vi "Top Level Launcher.vi"(6 "Variant in":variant, 7 "Shift Pressed?":bool, 8 "error in":errorcluster, 10 "QD Combo Box Ref":refnum<vi>, 11 "QD Launch VI Ref":refnum<vi>) -> (0 "error out":errorcluster, 4 "Variant out":variant)   [LabVIEW 2020]
doc: "Manages the top level VI in the project.\n\nNormal Operation:\nTo set the top VI, enter \"<b>s</b>\" or \"<b>set</b>\" before activating the shortcut.\nTo open the top VI, use Shift+Ctrl+[shortcut].\nTo run the top VI, use Ctrl+[shortcut].\n\nAdvanced Operation using QD data entry:\nTo run the top VI, enter \"r\" or \"run\" before activating the shortcut.\nTo remove the top VI setting, enter \"d\", \"del\", \"delete\", \"rem\", or \"remove\" before activating the shortcut.\nTo read what the top VI is, enter \"get\" or \"read\" before activating the shortcut.\nTo open the top VI without running it, enter \"o\" or \"open\" before activating the shortcut.\n\nDefault Shortcut - [E]"
panel:
  in  "Undo Name":string="Quick Drop Keyboard Shortcut"
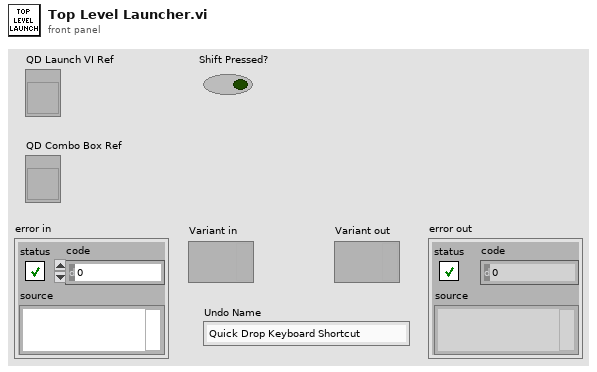
[diagram p1: front panel]
types:
  T1 = typedef "Command Enum.ctl" = enum16{"Invalid", "Invalid Alias", "Run", "Set", "Open", "Read", "Remove"}
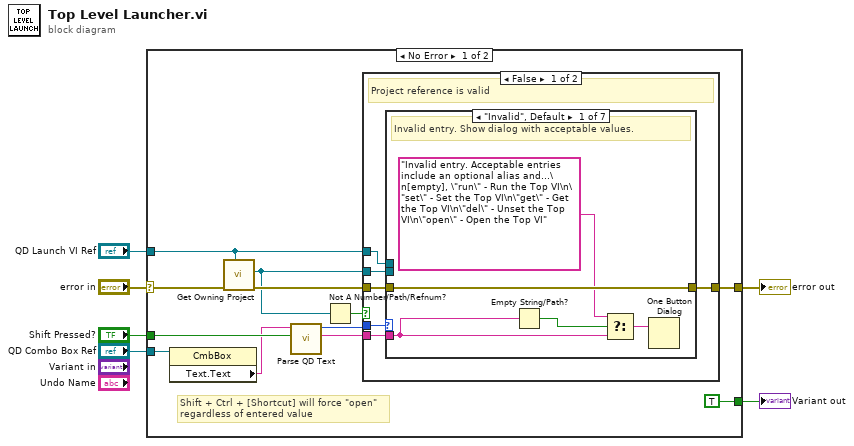
[diagram p0: block diagram]
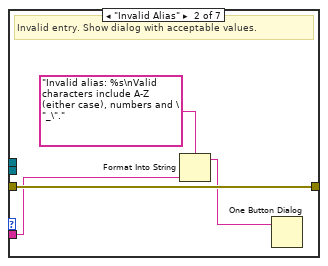
[diagram p2: hidden frame]
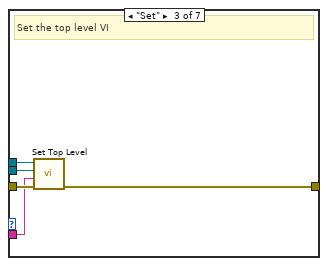
[diagram p3: hidden frame]
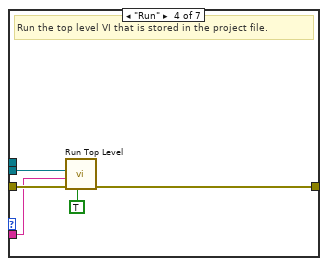
[diagram p4: hidden frame]
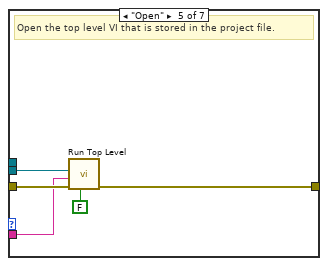
[diagram p5: hidden frame]
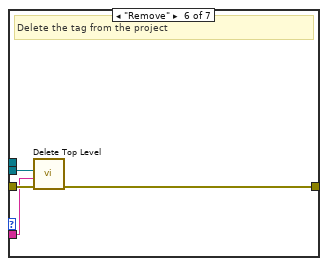
[diagram p6: hidden frame]
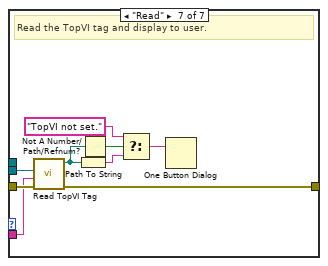
[diagram p7: hidden frame]
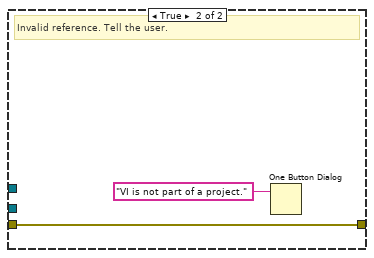
[diagram p8: hidden frame]
diagram:
  n1 = case shown="No Error" "error in" {
    selector: "error in" -> [w17 w64]
    tunnel: [w18 w64] -> w5
    tunnel: "QD Launch VI Ref" -> [w11 _]
    tunnel: "Shift Pressed?" -> [w9 _]
    tunnel: [TRUE _] -> w2
    tunnel: "QD Combo Box Ref" -> [w13 _]
    frame No Error {
      # "Shift + Ctrl + [Shortcut] will force \"open\"\nregardless of entered value"
      n2 = property class="CmbBox"(reference=w13) -> ("Text.Text"=w8:string)  [unwired: 1 in, 2 out]
      n3 = call "Get Owning Project.vi"("VI"=w11, "error in"=w17) -> ("error out"=w16:errorcluster, "Owning Project"=w12:refnum<vi>)  [unwired: 8 in]
      n4 = call "Parse QD Text.vi"("Shift Pressed?"=w9, "QD Combo Box Text"=w8) -> ("Parameter"=w7:string, "Command"=w10:T1)  [unwired: 8 in]
      n5 = Not A Number/Path/Refnum?(number/path/refnum=w12) -> (NaN/Path/Refnum?=w14:bool)
      n6 = case shown="False" w14 {
        tunnel: w10 -> [w22 _]
        tunnel: [w24 w63] -> w18
        tunnel: w16 -> [w23 w63]
        tunnel: w11 -> [w21 _]
        tunnel: w12 -> [w20 _]
        tunnel: w7 -> [w19 _]
        frame False {
          # "Project reference is valid"
          n7 = case shown="\"Invalid\", Default" w22 {
            tunnel: w23 -> [w29 w33 w38 w42 w47 w52 w61]
            tunnel: [w29 w33 w37 w43 w48 w51 w60] -> w24
            tunnel: w21 -> [_ _ w36 _ _ _ _]
            tunnel: w20 -> [_ _ w35 w41 w46 w50 w59]
            tunnel: w19 -> [w26 w31 w34 w39 w44 w49 w53]
            frame "Invalid", Default {
              # "Invalid entry. Show dialog with acceptable values."
              n8 = Empty String/Path?(string/path=w26) -> (empty?=w28:bool)
              n9 = Select(t="Invalid entry. Acceptable entries include an optional alias and...\n[empty], \"run\" - Run the Top VI\n\"set\" - Set the Top VI\n\"get\" - Get the Top VI\n\"del\" - Unset the Top VI\n\"open\" - Open the Top VI" ("message"), s=w28, f=w26) -> (s? t:f=w25:string)
              n10 = One Button Dialog(message=w25) -> ()  [unwired: 1 in, 1 out]
            }
            frame "Invalid Alias" {
              # "Invalid entry. Show dialog with acceptable values."
              n11 = Format Into String(format string="Invalid alias: %s\nValid characters include A-Z (either case), numbers and \"_\"." ("message"), w31) -> (resulting string=w30:string)  [unwired: 2 in, 1 out]
              n12 = One Button Dialog(message=w30) -> ()  [unwired: 1 in, 1 out]
            }
            frame "Set" {
              # "Set the top level VI"
              n13 = call "Set Top Level.vi"("error in"=w38, "Alias"=w34, "Project Reference"=w35, "VI Reference"=w36) -> ("error out"=w37:errorcluster)  [unwired: 7 in]
            }
            frame "Run" {
              # "Run the top level VI that is stored in the project file."
              n14 = call "Run Top Level.vi"("Run/Open (T = Run)"=TRUE ("Run/Open (F = Open)"), "error in"=w42, "Alias"=w39, "Project Reference"=w41) -> ("error out"=w43:errorcluster)  [unwired: 7 in]
            }
            frame "Open" {
              # "Open the top level VI that is stored in the project file."
              n15 = call "Run Top Level.vi"("Run/Open (T = Run)"=FALSE ("Run/Open (F = Open)"), "error in"=w47, "Alias"=w44, "Project Reference"=w46) -> ("error out"=w48:errorcluster)  [unwired: 7 in]
            }
            frame "Remove" {
              # "Delete the tag from the project"
              n16 = call "Delete Top Level.vi"("error in"=w52, "Alias"=w49, "Project Reference"=w50) -> ("error out"=w51:errorcluster)  [unwired: 8 in]
            }
            frame "Read" {
              # "Read the TopVI tag and display to user."
              n17 = call "Read TopVI Tag.vi"("error in"=w61, "Alias"=w53, "Project Reference"=w59) -> ("error out"=w60:errorcluster, "TopVI Path"=w58:path)  [unwired: 6 in, 1 out]
              n18 = Path To String(path=w58) -> (string=w56:string)
              n19 = Not A Number/Path/Refnum?(number/path/refnum=w58) -> (NaN/Path/Refnum?=w57:bool)
              n20 = Select(t="TopVI not set.", s=w57, f=w56) -> (s? t:f=w54:string)
              n21 = One Button Dialog(message=w54) -> ()  [unwired: 1 in, 1 out]
            }
          }
        }
        frame True {
          # "Invalid reference. Tell the user."
          n22 = One Button Dialog(message="VI is not part of a project.") -> ()  [unwired: 1 in, 1 out]
        }
      }
    }
    frame Error {
    }
  }
  "error out" <- w5
  "Variant out" <- w2
